vi "bats.parser.ip.vi"() -> ()   [LabVIEW 2022 SP3]
uses:
  data.ctl
  <vilib>/Platform/TimedLoop/XDataNode/timing_clust.ctl
  <vilib>/Platform/TimedLoop/XDataNode/nitl_modes.ctl
  <vilib>/Platform/TimedLoop/XDataNode/wakeup.ctl
  <vilib>/rvi/Emulation/niFpgaSctlEmulationGetInTimedLoop.vi
  <vilib>/rvi/Emulation/niFpgaEmulationReportErrorSimple.vi
  <vilib>/rvi/Emulation/niFpgaGetClockAttributes.vi
  <vilib>/rvi/Emulation/niFpgaCriticalErrorInLSC.vi
  <vilib>/rvi/Emulation/niFpgaEmulationIsFPGAContextNoSignature.vi
  <vilib>/rvi/errors/niFpgaSetErrorForExecOnDevCompSimple.vi
  <vilib>/rvi/eio/common/nirviEmuReportErrorAndStop.vi
  <vilib>/rvi/DataTransferAndStorage/Container/Common/niFpgaContainerGetUniqueNameForEmu.vi
  <vilib>/rvi/FIFO/Fifo_Resource/nirvififoEmulationSetSize.vi
  <vilib>/rvi/FIFO/Fifo_Resource/nirviFifoEmulationQueueMgr.vi
  <instcachedir>/0/nirviFifoEmulationQueueMgr_E5CAEC123FF24DC58D834DCA3CDAA9B5.lvgen/nirviFifoEmulationQueueMgr_E5CAEC123FF24DC58D834DCA3CDAA9B5_017.vi
  <vilib>/Utility/error.llb/Clear Errors.vi
  <vilib>/rvi/FIFO/Fifo_Resource/nirvififoEmulationCreateLock.vi
  <vilib>/rvi/Emulation/niFpgaProcessEmulError.vi
  <vilib>/rvi/FIFO/Fifo_Resource/nirvififoEmulationObtainLock.vi
  <vilib>/rvi/FIFO/Fifo_Resource/nirvififoEmulationReleaseLock.vi
  <vilib>/rvi/occurrence/nirviWaitOnOccurrenceBase.vi
  <vilib>/rvi/errors/nirviReportUnexpectedCaseInternalError.vi
  <vilib>/rvi/errors/nirviReportUnexpectedCaseInternalError (U32).vi
  <instcachedir>/0/nirviFifoEmulationQueueMgr_E5CAEC123FF24DC58D834DCA3CDAA9B5.lvgen/nirviFifoEmulationQueueMgr_E5CAEC123FF24DC58D834DCA3CDAA9B5_000.vi
  <vilib>/Platform/TimedLoop/XDataNode/XDataNode.xnode
  <vilib>/rvi/DataTransferAndStorage/Container/XNode/niFpgaContainer.xnode
  <vilib>/rvi/FIFO/Fifo_Resource/nirvififoEmulationRead.vi
  <vilib>/Platform/TimedLoop/XDataNode/XDNodeRunTimeDep.lvlib
panel:
  out "OrderBook Command.Type":T1(ring)
  out "Debug.Valid":bool
  out "Debug.Element":u64
  in  "Ready.For.Debug":bool
  in  "data":T2={"enabled"=[FALSE, FALSE, FALSE, FALSE, FALSE, FALSE, FALSE, FALSE], "byte"=[0, 0, 0, 0, 0, 0, 0, 0]} {"byte" format="%.0x"}
  out "OrderBook.Command.Valid":bool
  out "Cancelled Quantity (U32)":u32
  out "Executed Quantity (U32)":u32
  out "Price (U64)":u64
  out "Symbol (U64)":u64
  out "Quantity (U32)":u32
  out "Order Id (U64)":u64
  out "Side (U8)":u8
  in  "Ready.for.OrderBook.Command":bool
  out "Ready.for.Udp.Input":bool
  in  "data.valid":bool
  in  "reset":bool
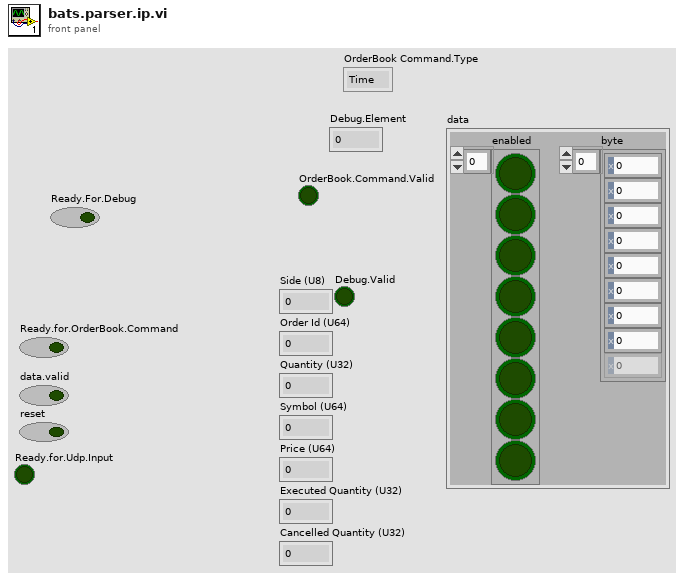
[diagram p1: front panel]
types:
  T1 = enum16{"Time", "AddOrder", "OrderExecuted", "OrderExecutedAtPrice", "ReduceSize", "ModifyOrder", "DeleteOrder", "Get.All.Orders", "Get.Top"}
  T2 = typedef "data.ctl" = cluster{"enabled":bool[], "byte":u8[]}
  T3 = typedef "XDNodeRunTimeDep.lvlib/timing_clust.ctl" = cluster{"Expected End [f-1]":u64, "Actual End [f-1]":u64, "Finished Late? [f-1]":bool, "Expected End [i-1]":u64, "Actual End [i-1]":u64, "Finished Late? [i-1]":bool, "Expected Start [i]":u64, "Actual Start [i]":u64, "Expected Start [f]":u64, "Actual Start [f]":u64, "Source Name":string, "Structure Name":string, "Period":i64, "Deadline":i64, "Offset":i64, "Start":i64, "Priority":i32, "Timeout":i32, "Mode":T4, "Wakeup Reason":T5, "Error":errorcluster, "Source Type":string, "Secondary Source Type":string, "Global End Time":u64, "Global Start Time":u64, "Frame Duration":u64, "Iteration Duration":u64, "Assigned CPU":i32, "I/O Scan Engine Mode":u32}
  T4 = typedef "XDNodeRunTimeDep.lvlib/nitl_modes.ctl" = enum32{"No Change", "Process missed periods, maintain original phase", "Discard missed periods, maintain original phase", "Process missed periods, ignore original phase", "Discard missed periods, ignore original phase"}
  T5 = typedef "XDNodeRunTimeDep.lvlib/wakeup.ctl" = enum32{"Normal", "Aborted", "Asynchronous wakeup", "Timing source error", "Timed loop error", "Timeout"}
  T6 = cluster{"OrderBook Command.Type":enum16{"Time", "AddOrder", "OrderExecuted", "OrderExecutedAtPrice", "ReduceSize", "ModifyOrder", "DeleteOrder", "Get.All.Orders", "Get.Top"}, "Side (U8)":u8, "Order Id (U64)":u64, "Quantity (U32)":u32, "Symbol (U64)":u64, "Price (U64)":u64, "Executed Quantity (U32)":u32, "Canceled Quantity (U32)":u32, "Remaining Quantity (U32)":u32, "Seconds (U64)":u64, "Nanoseconds (U64)":u64}
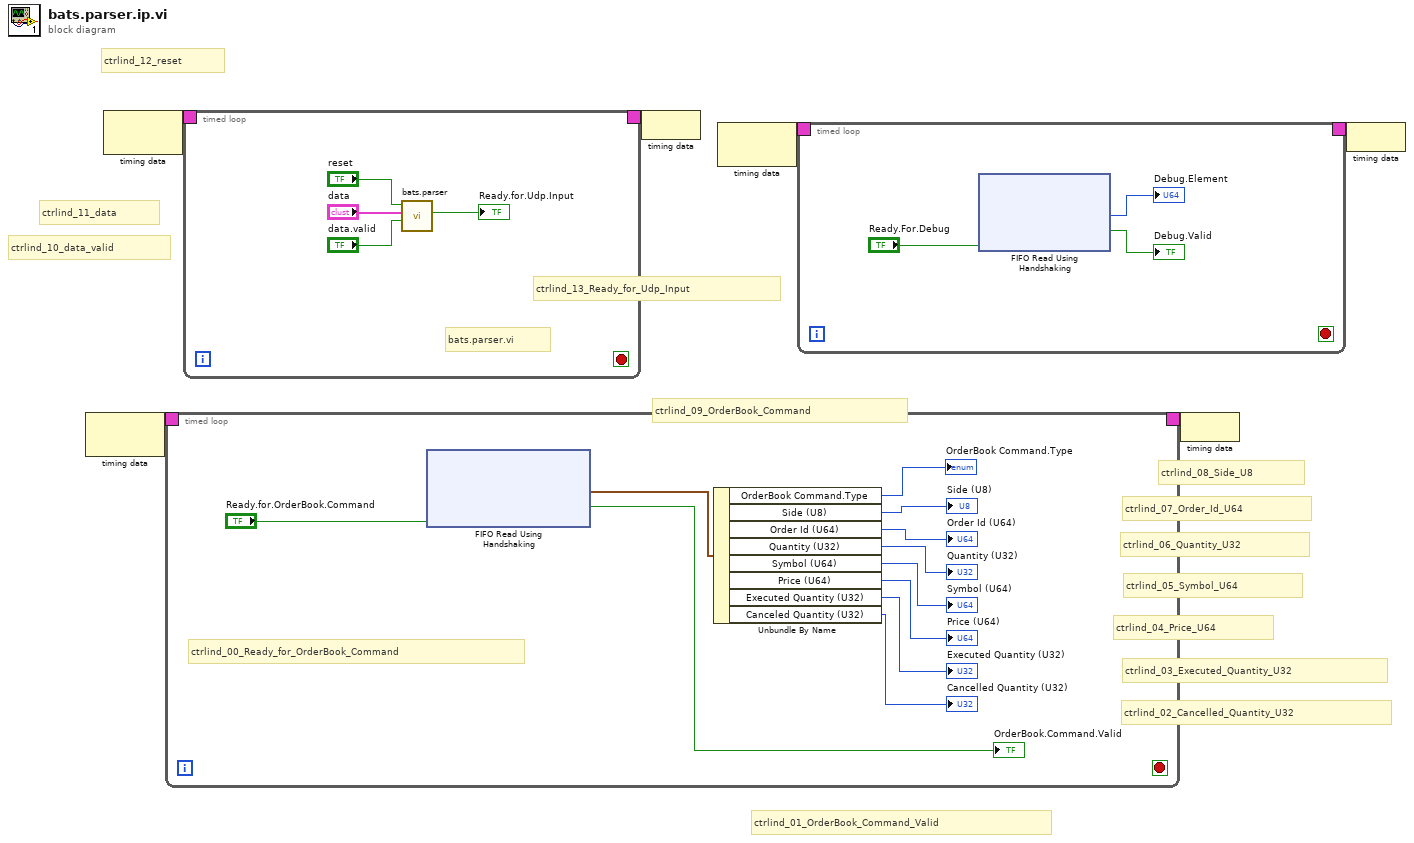
[diagram p0: block diagram]
diagram:
  # "ctrlind_09_OrderBook_Command"
  # "ctrlind_08_Side_U8"
  # "ctrlind_07_Order_Id_U64"
  # "ctrlind_06_Quantity_U32"
  # "ctrlind_05_Symbol_U64"
  # "ctrlind_04_Price_U64"
  # "ctrlind_03_Executed_Quantity_U32"
  # "ctrlind_02_Cancelled_Quantity_U32"
  # "ctrlind_01_OrderBook_Command_Valid"
  # "ctrlind_13_Ready_for_Udp_Input"
  # "ctrlind_11_data"
  # "ctrlind_10_data_valid"
  # "ctrlind_12_reset"
  n1 = node-c288() -> (w4:T3)  [unwired: 1 in]
  n2 = node-c288() -> (w6:T3)  [unwired: 1 in]
  n3 = timed-loop {
    timing: w4 -> [_]
    timing-out: [_] -> w3
    stop <- _ stop-if-true
    # "ctrlind_00_Ready_for_OrderBook_Command"
    n4 = xnode ("FIFO Read Using Handshaking")("Ready for Output"="Ready.for.OrderBook.Command") -> ("Element"=w10:T6, "Output Valid"=→"OrderBook.Command.Valid":bool)  [unwired: 1 in, 1 out]
    n5 = Unbundle By Name(w10) -> ("OrderBook Command.Type"=→"OrderBook Command.Type":T1, "Side (U8)"=→"Side (U8)":u8, "Order Id (U64)"=→"Order Id (U64)":u64, "Quantity (U32)"=→"Quantity (U32)":u32, "Symbol (U64)"=→"Symbol (U64)":u64, "Price (U64)"=→"Price (U64)":u64, "Executed Quantity (U32)"=→"Executed Quantity (U32)":u32, "Canceled Quantity (U32)"=→"Cancelled Quantity (U32)":u32)
  }
  n6 = timed-loop {
    timing: w6 -> [_]
    timing-out: [_] -> w5
    stop <- _ stop-if-true
    # "bats.parser.vi"
    n7 = call "bats.parser.vi"("data.valid"="data.valid", "data"="data", "reset"="reset") -> ("Ready.for.Udp.Input"=→"Ready.for.Udp.Input":bool)  [unwired: 8 in]
  }
  n8 = node-c288(w5) -> ()
  n9 = node-c288() -> (w2:T3)  [unwired: 1 in]
  n10 = timed-loop {
    timing: w2 -> [_]
    timing-out: [_] -> w1
    stop <- _ stop-if-true
    n11 = xnode ("FIFO Read Using Handshaking")("Ready for Output"="Ready.For.Debug") -> ("Element"=→"Debug.Element":u64, "Output Valid"=→"Debug.Valid":bool)  [unwired: 1 in, 1 out]
  }
  n12 = node-c288(w3) -> ()
  n13 = node-c288(w1) -> ()
